vi "List Principal Policies.vi"(8 "error in (no error)":errorcluster, 10 "Principal":string, 11 "IoT Session in":refnum<class "IoT Session.lvclass">) -> (0 "error out":errorcluster, 2 "Principal Policies":string[](array[string]), 3 "IoT Session out":refnum<class "IoT Session.lvclass">)   [LabVIEW 2015, in "NI_AWS_IoT.lvlib" / "IoT Session.lvclass"]
uses:
  IoT Session.lvclass
  Core/HTTP Request/Request Options.ctl
  Core/HTTP Request/Name Value Pair.ctl
  Core/HTTP Request/Region handling.ctl
  Core/HTTP Request/URL formatting.ctl
  Core/HTTP Request/HTTP Request.lvclass
  JSON Parsing/NI_JSON Parsing.lvlib
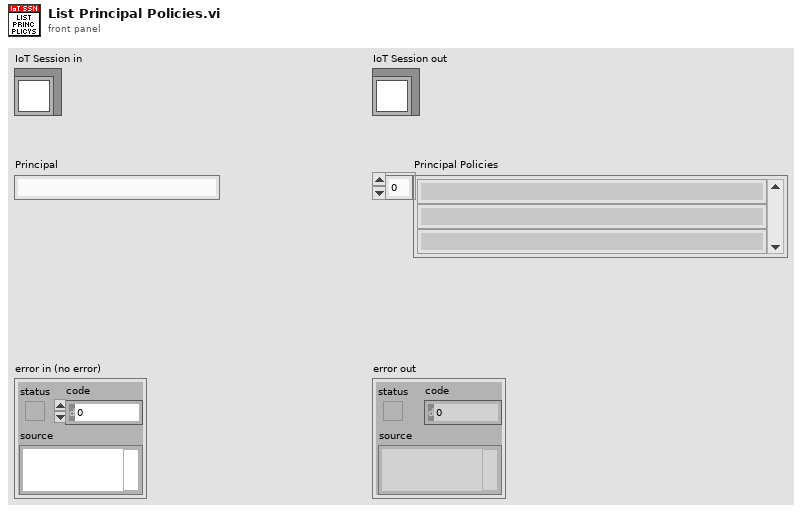
[diagram p1: front panel]
types:
  T1 = typedef "NI_AWS_Core.lvlib/HTTP Request.lvclass/Name Value Pair.ctl" = cluster{"name":string, "value":string}
  T2 = typedef "NI_AWS_Core.lvlib/HTTP Request.lvclass/Request Options.ctl" = cluster{"request headers":T1[], "request parameters":T1[], "request body":string, "region handling":T3, "URL formatting":T4}
  T3 = typedef "NI_AWS_Core.lvlib/HTTP Request.lvclass/Region handling.ctl" = enum16{"use region everywhere", "use region (authentication only)", "use region (URL only)", "ignore region everwhere"}
  T4 = typedef "NI_AWS_Core.lvlib/HTTP Request.lvclass/URL formatting.ctl" = enum16{"region-", "region."}
  T5 = typedef "NI_AWS_Core.lvlib/HTTP Request.lvclass/Response.ctl" = cluster{"Headers":string, "Body":string}
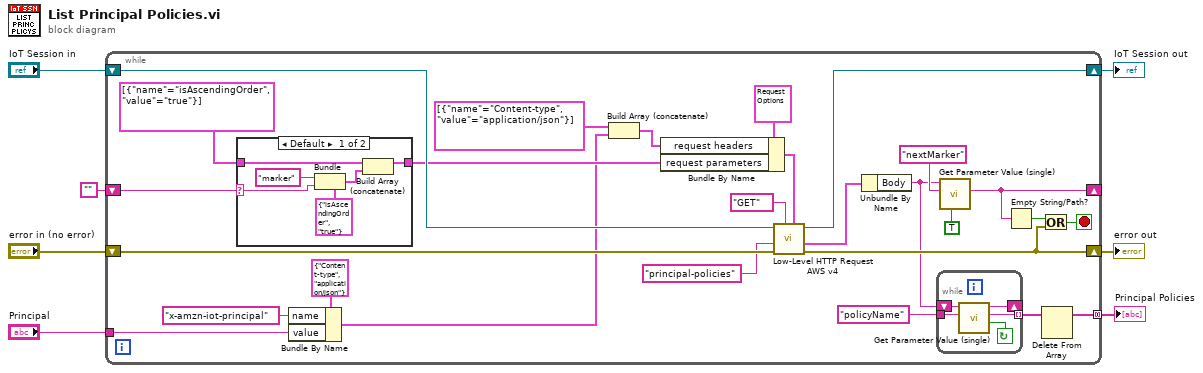
[diagram p0: block diagram]
diagram:
  n1 = while {
    shift-right: [w22] -> w6
    shift-left: "error in (no error)" -> [w31]
    shift-right: [w30] -> w5
    shift-left: "IoT Session in" -> [w29]
    shift-right: [w24] -> _
    shift-left: "" -> [w26]
    tunnel: [w8] -> w2 mode=concatenating
    tunnel: "Principal" -> [w12]
    stop <- w21 stop-if-true
    n2 = case shown="Default" w26 {
      selector: w26 -> [w41 _]
      tunnel: T1[] [{"name"="isAscendingOrder", "value"="true"}] ("request parameters") -> [w45 w46]
      tunnel: [w44 w46] -> w16
      frame Default {
        n3 = Bundle(cluster=T1 {"name"="isAscendingOrder", "value"="true"} ("Name Value Pair"), "name"="marker", "value"=w41) -> (w42:T1)
        n4 = Build Array (concatenate)(w45, w42) -> (w44:T1[])
      }
      frame "" {
      }
    }
    n5 = Bundle By Name(cluster=T1 {"name"="Content-type", "value"="application/json"} ("Cluster"), "name"="x-amzn-iot-principal", "value"=w12) -> (w11:T1)
    n6 = Build Array (concatenate)(T1[] [{"name"="Content-type", "value"="application/json"}] ("request headers"), w11) -> (w15:T1[])
    n7 = Bundle By Name(cluster=T2 {"request headers"=[], "request parameters"=[], "request body"="", "region handling"=enum."use region everywhere", "URL formatting"=enum."region."} ("Request Options"), "request headers"=w15, "request parameters"=w16) -> (w32:T2)
    n8 = call "Low-Level HTTP Request AWS v4.vi"("Request Options"=w32, "HTTP-Verb"="GET", "error in (no error)"=w31, "URL Suffix"="principal-policies" ("string"), "AWS Core in"=w29) -> ("error out"=w22:errorcluster, "Response"=w27:T5, "AWS Core out"=w30:refnum<class "IoT Session.lvclass">)  [unwired: 3 in, 1 out]
    n9 = Unbundle By Name(w27) -> ("Body"=w10:string)
    n10 = while {
      tunnel: "policyName" ("Parameter Name") -> [w39]
      tunnel: [w38] -> w9 mode=indexing
      shift-right: [w36] -> _
      shift-left: w10 -> [w37]
      stop <- w35 continue-if-true
      n11 = call "Get Parameter Value (single).vi"("Parameter Name"=w39, "JSON"=w37) -> ("Found"=w35:bool, "Parameter Value"=w38:string, "Remaining JSON"=w36:string)  [unwired: 6 in, 1 out]
    }
    n12 = call "Get Parameter Value (single).vi"("Clear Null"=TRUE, "Parameter Name"="nextMarker", "JSON"=w10) -> ("Parameter Value"=w24:string)  [unwired: 5 in, 3 out]
    n13 = Empty String/Path?(string/path=w24) -> (empty?=w23:bool)
    n14 = Or(x=w23, y=w22) -> (x .or. y?=w21:bool)
    n15 = Delete From Array(array=w9) -> (array with subset deleted=w8:string[])  [unwired: 2 in, 1 out]
  }
  "error out" <- w6
  "IoT Session out" <- w5
  "Principal Policies" <- w2
